vi "MesGetProductInfo.vi"(8 "error in":errorcluster, 9 "设备码":string="gmt_create", 10 "托盘编码值":string="d7", 11 "connection reference":T1) -> (0 "error out":errorcluster, 1 "加工状态":string[](array[string]), 3 "错误状态":bool)   [LabVIEW 2014]
uses:
  <vilib>/addons/database/Connection.llb/Conn ObjectReference.ctl
  <vilib>/addons/database/Auxilliary.llb/DB Tools Parameter Info.ctl
  <vilib>/addons/database/Auxilliary.llb/DB Tools DataTypes.ctl
  <vilib>/addons/database/Auxilliary.llb/DB Tools Parameter Dir.ctl
  <vilib>/addons/database/Connection.llb/DB Tools Open Connec (String).vi
  <vilib>/addons/database/Command.llb/Cmd Set Parameter Value (C).vi
  <vilib>/addons/database/Command.llb/Cmd Execute.vi
  <vilib>/addons/database/Recordset.llb/Rec Fetch Recordset Data (CR).vi
  <vilib>/addons/database/Recordset.llb/Rec Destroy - Command.vi
  <vilib>/addons/database/_DB Variant To Data/Database Variant To Data.xnode
  <vilib>/addons/database/NI_Database_API.lvlib
panel:
  out "查找的结果":string[][](array[string])
  out "recordset data":variant[][](array[variant])
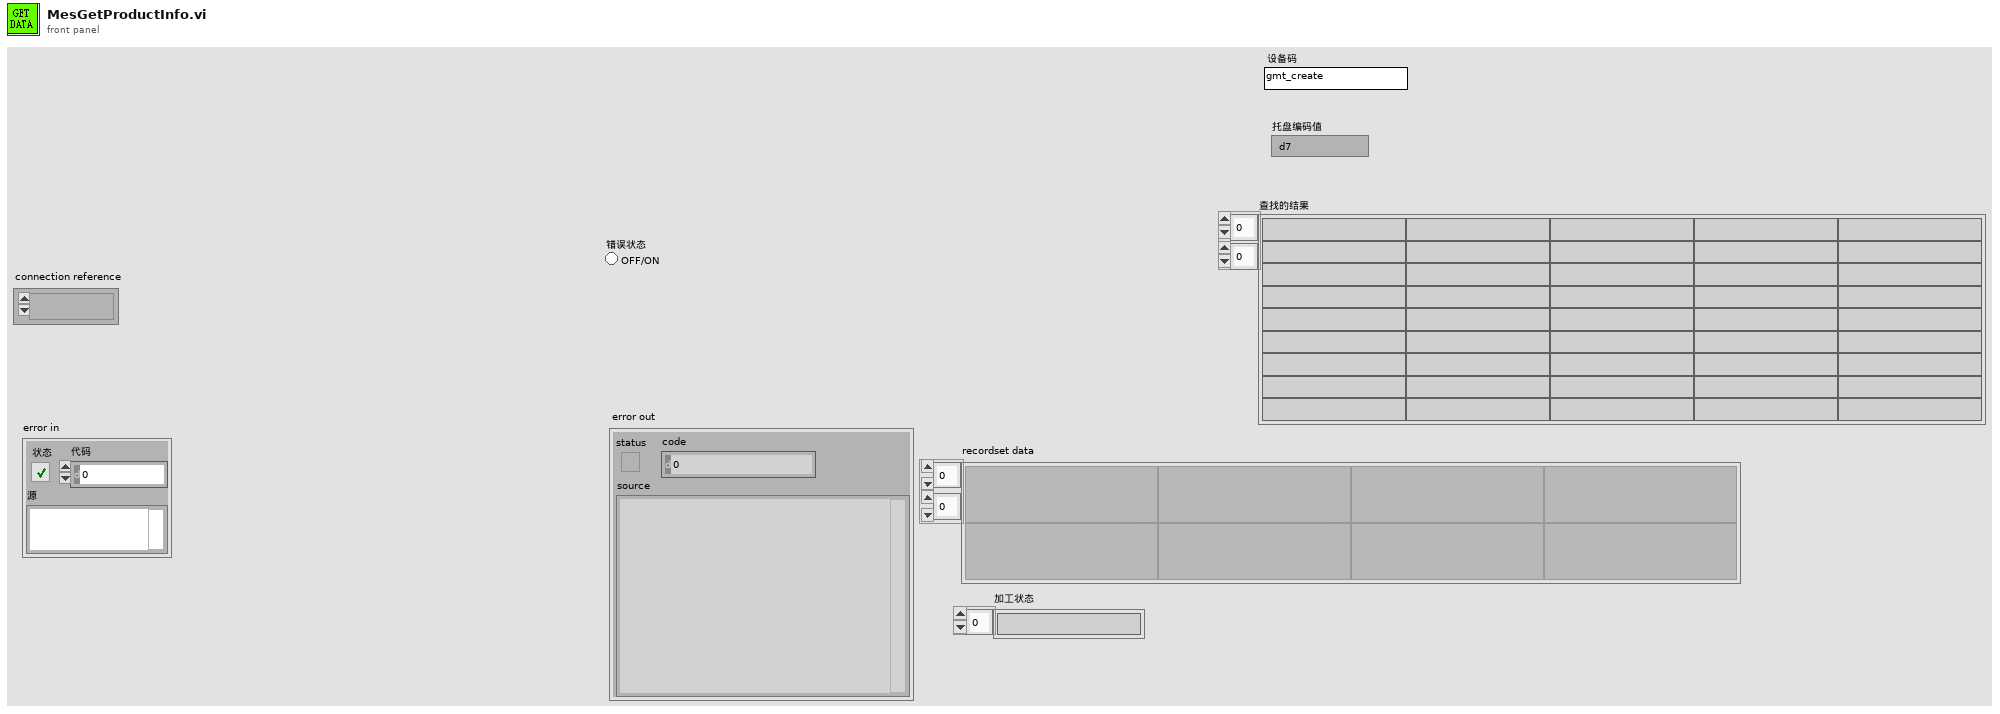
[diagram p1: front panel]
types:
  T1 = typedef "NI_Database_API.lvlib/Conn ObjectReference.ctl" = refnum<k1>
  T2 = typedef "NI_Database_API.lvlib/DB Tools Parameter Info.ctl" = cluster{"parameter name":string, "type":T3, "direction":T4, "value":variant}
  T3 = typedef "NI_Database_API.lvlib/DB Tools DataTypes.ctl" = enum16{"String", "Long (I32)", "Single (SGL)", "Double (DBL)", "Date/Time", "Binary"}
  T4 = typedef "NI_Database_API.lvlib/DB Tools Parameter Dir.ctl" = enum32{"Input", "Output", "Input/Output", "Return Value"}
  T5 = typedef "NI_Database_API.lvlib/Cmd ObjectReference.ctl" = refnum<k1>
  T6 = typedef "NI_Database_API.lvlib/Cmd-Rec Object Reference.ctl" = refnum<k1>
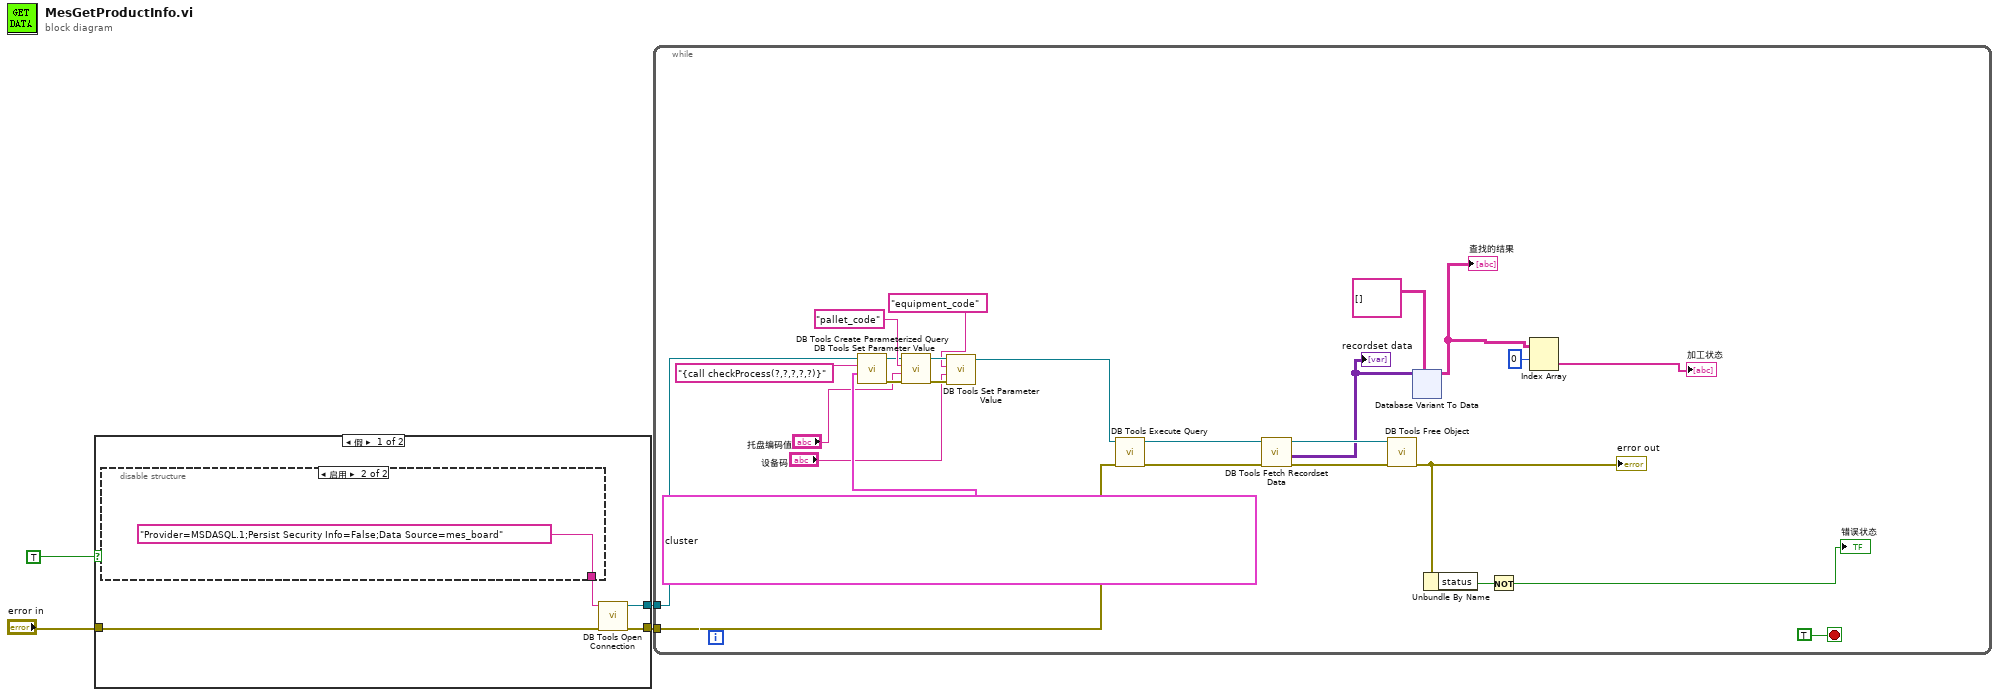
[diagram p0: block diagram]
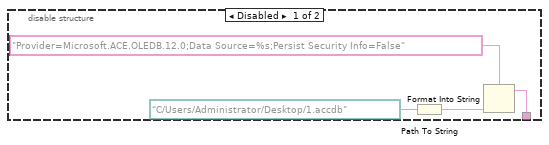
[diagram p2: hidden frame]
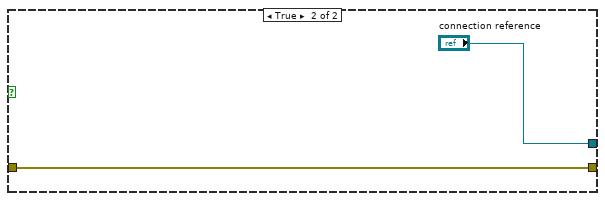
[diagram p3: hidden frame]
diagram:
  n1 = case shown="假" TRUE {
    tunnel: [w8 "connection reference"] -> w2
    tunnel: [w7 w14] -> w3
    tunnel: "error in" -> [w5 w14]
    frame False {
      n2 = disable-structure shown="启用" {
        disable-tunnel: [w11 "Provider=MSDASQL.1;Persist Security Info=False;Data Source=mes_board" ("connection information")] -> w6
        frame Disabled {
          n3 = Path To String(path=path "C:/Users/Administrator/Desktop/1.accdb" ("路径")) -> (string=w12:string)
          n4 = Format Into String(format string="Provider=Microsoft.ACE.OLEDB.12.0;Data Source=%s;Persist Security Info=False" ("初始字符串"), w12) -> (resulting string=w11:string)  [unwired: 2 in, 1 out]
        }
        frame Enabled {
        }
      }
      n5 = call-poly <vilib>:"DB Tools Open Connection.vi"("error in (no error)"=w5, "connection information"=w6) -> ("error out"=w7:errorcluster, "connection reference"=w8:T1)  [unwired: 6 in]
    }
    frame True {
    }
  }
  n6 = while {
    tunnel: w2 -> [w23]
    tunnel: w3 -> [w39]
    stop <- TRUE stop-if-true
    n7 = call <vilib>:"DB Tools Create Parameterized Query.vi"("parameters"=T2[] [{"parameter name"="msg_code", "type"=enum."String", "direction"=enum."Output", "value"=variant}, {"parameter name"="msg", "type"=enum."String", "direction"=enum."Output", "value"=variant}, {"parameter name"="product", "type"=enum."String", "direction"=enum."Output", "value"=variant}, {"parameter name"="pallet_code", "type"=enum."String", "direction"=enum."Input", "value"=variant}, {"parameter name"="equipment_code", "type"=enum."String", "direction"=enum."Input", "value"=variant}], "SQL query"="{call checkProcess(?,?,?,?,?)}", "connection reference"=w23) -> ("error out"=w25:errorcluster, "command reference"=w24:T5)  [unwired: 4 in, 1 out]
    n8 = call-poly <vilib>:"DB Tools Set Parameter Value.vi"("error in (no error)"=w25, "value"="托盘编码值", "parameter index"="pallet_code", "command reference"=w24) -> ("error out"=w21:errorcluster, "command reference out"=w22:T5)  [unwired: 4 in]
    n9 = call-poly <vilib>:"DB Tools Set Parameter Value.vi"("error in (no error)"=w21, "value"="设备码", "parameter index"="equipment_code", "command reference"=w22) -> ("command reference out"=w16:T5)  [unwired: 4 in, 1 out]
    n10 = call-poly <vilib>:"DB Tools Execute Query.vi"("error in (no error)"=w39, "command reference"=w16) -> ("error out"=w38:errorcluster, "command-recordset reference"=w33:T6)  [unwired: 6 in]
    n11 = call-poly <vilib>:"DB Tools Fetch Recordset Data.vi"("error in (no error)"=w38, "command-recordset reference"=w33) -> ("error out"=w37:errorcluster, "recordset data"=w35:variant[][], "command-recordset reference out"=w36:T6)  [unwired: 3 in]
    "recordset data" <- w35
    n12 = call-poly <vilib>:"DB Tools Free Object.vi"("error in (no error)"=w37, "command-recordset reference"=w36) -> ("error out"=w32:errorcluster)  [unwired: 8 in, 1 out]
    "error out" <- w32
    n13 = xnode "Database Variant To Data"("database variant"=w35, "type"=string[][] [] ("columns")) -> ("data"=w30:string[][])  [unwired: 1 in, 1 out]
    "查找的结果" <- w30
    n14 = Unbundle By Name(w32) -> ("status"=w41:bool)
    n15 = Not(x=w41) -> (.not. x?=→"错误状态":bool)
    n16 = Index Array(array=w30, index (row)=0 ("索引 (行)")) -> (element=→"加工状态":string[])  [unwired: 1 in]
  }
